vi "IMcalc.vi"(5 "F2":dbl, 6 "F1":dbl) -> (1 "LIM":dbl, 2 "UIM":dbl)   [LabVIEW 2018]
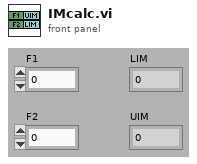
[diagram p1: front panel]
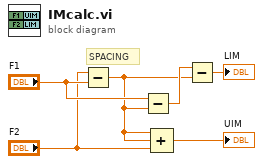
[diagram p0: block diagram]
diagram:
  # "SPACING"
  n1 = Subtract(x="F2", y="F1") -> (x-y=w3:dbl)
  n2 = Subtract(x="F1", y=w3) -> (x-y=w5:dbl)
  n3 = Compound Arithmetic op=ADD(w3, w3, "F2") -> (→"UIM":dbl)
  n4 = Subtract(x=w5, y=w3) -> (x-y=→"LIM":dbl)
